vi "Measurement UI.vi"() -> ()   [LabVIEW 2020]
panel:
  out "xy data out":cluster{"x_data":dbl[], "y_data":dbl[]}(graph)
  out "u32 animal enum out":enum32{"Rabbit", "Gopher", "Badger"}(ring)=enum."Badger"
  out "u32 color ring out":u32(ring)=2 items=["Red", "Green", "Blue"]
  out "string out":string="Empty"
  out "bool out":bool
  out "I64 out":i64
  out "I64 array out":i64[](array[numeric])
  out "I32 out":i32
  out "I32 array out":i32[](array[numeric])
  out "U64 out":u64
  out "U64 array out":u64[](array[numeric])
  out "U32 out":u32
  out "U32 array out":u32[](array[numeric])
  out "double out":dbl
  out "double array out":dbl[](array[numeric])
  in  "u32 animal enum in":enum32{"Rabbit", "Gopher", "Badger"}(ring)
  in  "u32 color ring in":u32(ring) items=["Red", "Green", "Blue"]
  in  "string in":string
  in  "bool in":bool
  in  "I64 in":i64
  in  "I64 array in":i64[](array[numeric])
  in  "I32 in":i32
  in  "I32 array in":i32[](array[numeric])
  in  "U64 in":u64
  in  "U64 array in":u64[](array[numeric])
  in  "U32 in":u32
  in  "U32 array in":u32[](array[numeric])
  in  "double in":dbl
  in  "double array in":dbl[](array[numeric])
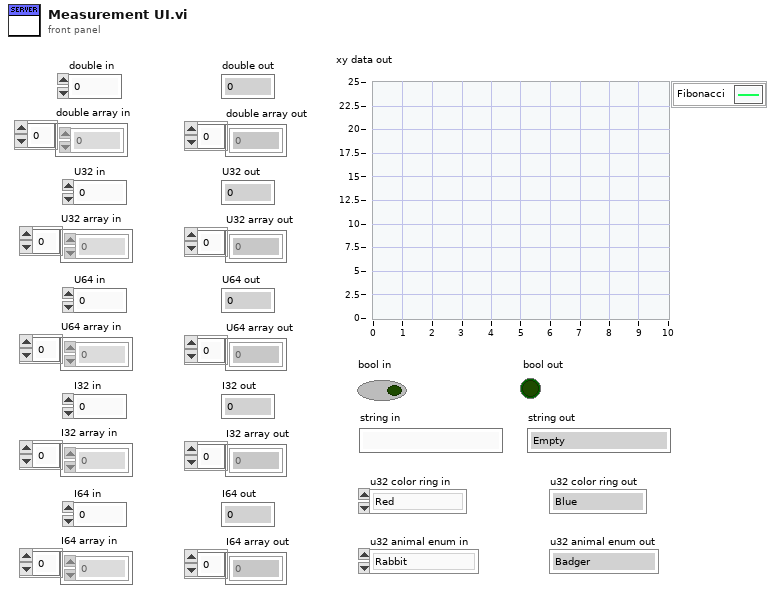
[diagram p1: front panel]
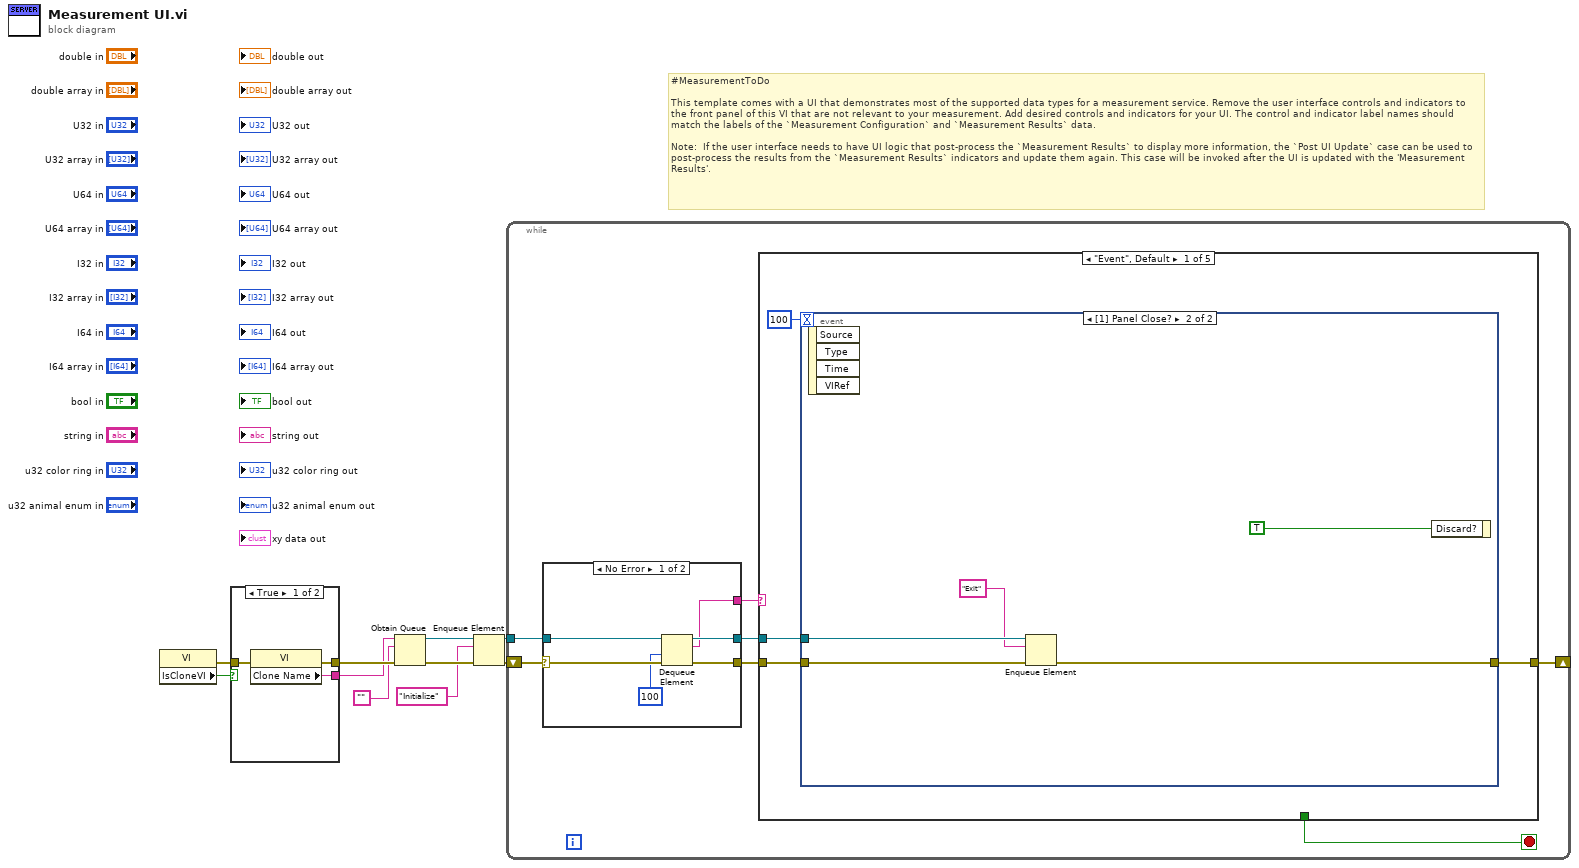
[diagram p0: block diagram]
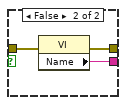
[diagram p2: hidden frame]
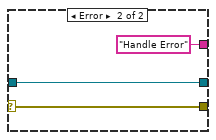
[diagram p3: hidden frame]
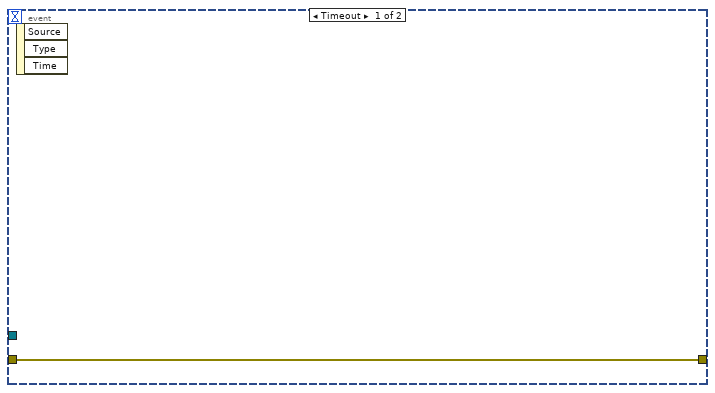
[diagram p4: hidden frame]
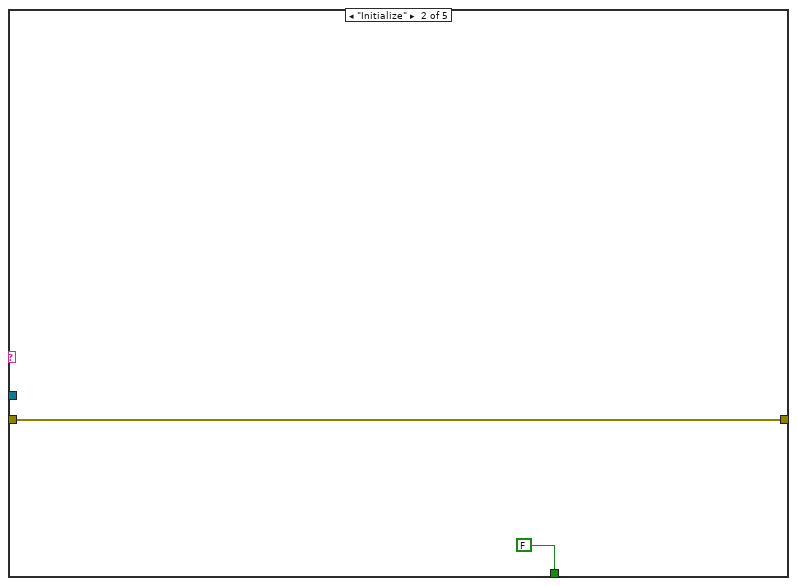
[diagram p5: hidden frame]
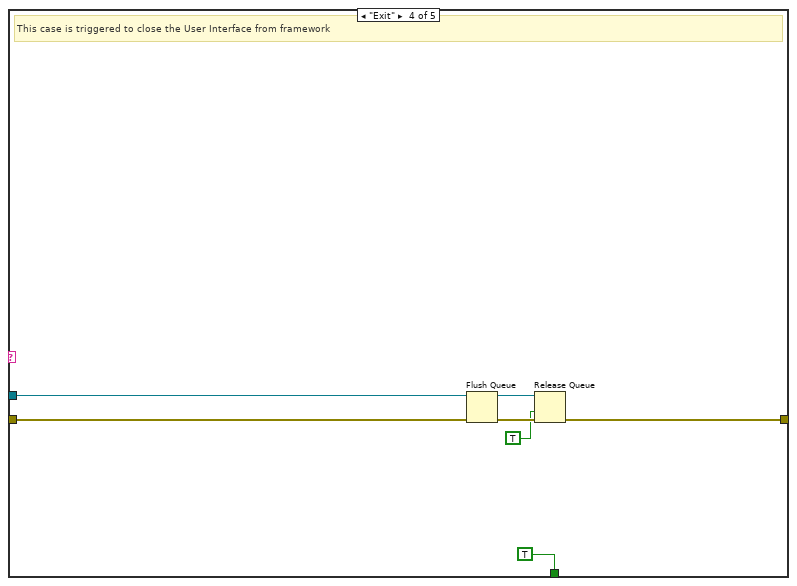
[diagram p7: hidden frame]
diagram:
  # "#MeasurementToDo  \n\nThis template comes with a UI that demonstrates most of the supported data types for a measurement service. Remove the user interface controls and indicators to the front panel of this VI that are not relevant to your measurement. Add desired controls and indicators for your UI. The control and indicator label names should match the labels of the `Measurement Configuration` and `Measurement Results` data.\n\nNote:  If the user interface needs to have UI logic that post-process the `Measurement Results` to display more information, the `Post UI Update` case can be used to post-process the results from the `Measurement Results` indicators and update them again. This case will be invoked after the UI is updated with the 'Measurement Results'."
  n1 = property class="VI"() -> (error out=w1:errorcluster, "IsCloneVI"=w2:bool)  [unwired: 2 in, 1 out]
  n2 = case shown="True" w2 {
    tunnel: [w13 w16] -> w10
    tunnel: [w12 w15] -> w9
    tunnel: w1 -> [w11 w14]
    frame True {
      n3 = property class="VI"(error in=w11) -> (error out=w13:errorcluster, "Clone Name"=w12:string)  [unwired: 1 in, 1 out]
    }
    frame False {
      n4 = property class="VI"(error in=w14) -> (error out=w16:errorcluster, "Name"=w15:string)  [unwired: 1 in, 1 out]
    }
  }
  n5 = Obtain Queue(name (unnamed)=w9, element data type="", error in (no error)=w10) -> (queue out=w6:refnum<queue>, error out=w8:errorcluster)  [unwired: 2 in, 1 out]
  n6 = Enqueue Element(queue=w6, element="Initialize", error in (no error)=w8) -> (queue out=w5:refnum<queue>, error out=w7:errorcluster)  [unwired: 1 in, 1 out]
  n7 = while {
    shift-right: [w18] -> _
    shift-left: w7 -> [w23]
    tunnel: w5 -> [w21]
    stop <- w17 stop-if-true
    n8 = case shown="No Error" w23 {
      selector: w23 -> [w29 w32]
      tunnel: [w28 w32] -> w22
      tunnel: w21 -> [w27 w31]
      tunnel: [w26 w31] -> w20
      tunnel: [w25 "Handle Error"] -> w19
      frame No Error {
        n9 = Dequeue Element(queue=w27, timeout in ms (-1)=100, error in (no error)=w29) -> (queue out=w26:refnum<queue>, element=w25:string, error out=w28:errorcluster)  [unwired: 1 out]
      }
      frame Error {
      }
    }
    n10 = case shown="\"Event\", Default" w19 {
      tunnel: w22 -> [w35 w44 w45 w52 w53]
      tunnel: w20 -> [w33 _ _ w50 _]
      tunnel: [w36 w44 w45 w47 w53] -> w18
      tunnel: [_ FALSE _ TRUE _] -> w17
      frame "Event", Default {
        n11 = event shown="[1] Panel Close?" {
          selector: _ -> [_ _]
          dyn-events: _ -> [_ _]
          timeout: 100 -> [_ _]
          tunnel: [w37 w40] -> w36
          tunnel: w35 -> [w37 w41]
          tunnel: w33 -> [_ w39]
          event Timeout {
            n12 = event-data() -> ()  [unwired: 1 in, 3 out]
          }
          event Panel Close? {
            n13 = event-data() -> ()  [unwired: 1 in, 4 out]
            n14 = Enqueue Element(queue=w39, element="Exit", error in (no error)=w41) -> (error out=w40:errorcluster)  [unwired: 1 in, 2 out]
            n15 = event-data("Discard?"=TRUE) -> ()  [unwired: 1 in, 1 out]
          }
        }
      }
      frame "Initialize" {
      }
      frame "Post UI Update" {
        # "This case will be triggered, after framework updates the User interface with result values."
      }
      frame "Exit" {
        # "This case is triggered to close the User Interface from framework"
        n16 = Flush Queue(queue=w50, error in (no error)=w52) -> (queue out=w49:refnum<queue>, error out=w48:errorcluster)  [unwired: 1 out]
        n17 = Release Queue(queue=w49, force destroy? (F)=TRUE, error in (no error)=w48) -> (error out=w47:errorcluster)  [unwired: 2 out]
      }
      frame "Handle Error" {
      }
    }
  }
